vi "datahandle.vi"(8 "error in (no error)":errorcluster caption="错误输入（无错误）", 10 "data":string[][](array[string]), 11 "HJ212 输入":refnum<class "HJ212.lvclass">) -> (0 "error out":errorcluster caption="错误输出", 2 "message":string, 3 "HJ212 输出":refnum<class "HJ212.lvclass">)   [LabVIEW 2016, in "中水三立SQL数据传输.lvlib" / "HJ212.lvclass"]
uses:
  HJ212.lvclass
  data_combination/data_combination.lvclass/data_combination.ctl
  data_combination/data_combination.lvclass
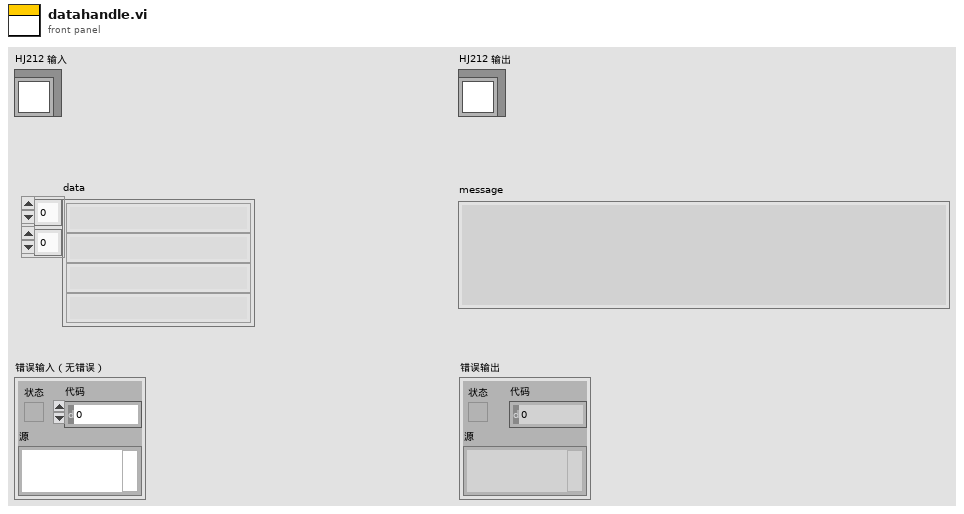
[diagram p1: front panel]
types:
  T1 = cluster{"请求编码QN(20)":string, "系统编码ST(5)":string, "命令编码CN(7)":string, "访问密码PW(9)":string, "设备唯一标识MN(27)":string, "拆分包及应答标志FLAG(8)":string, "总包数PNUM(9)":string, "包号PNO(8)":string, "指令参数CP(0-950)":string}
  T2 = typedef "中水三立SQL数据传输.lvlib/table.ctl" = string
  T3 = typedef "中水三立SQL数据传输.lvlib/Type.ctl" = string
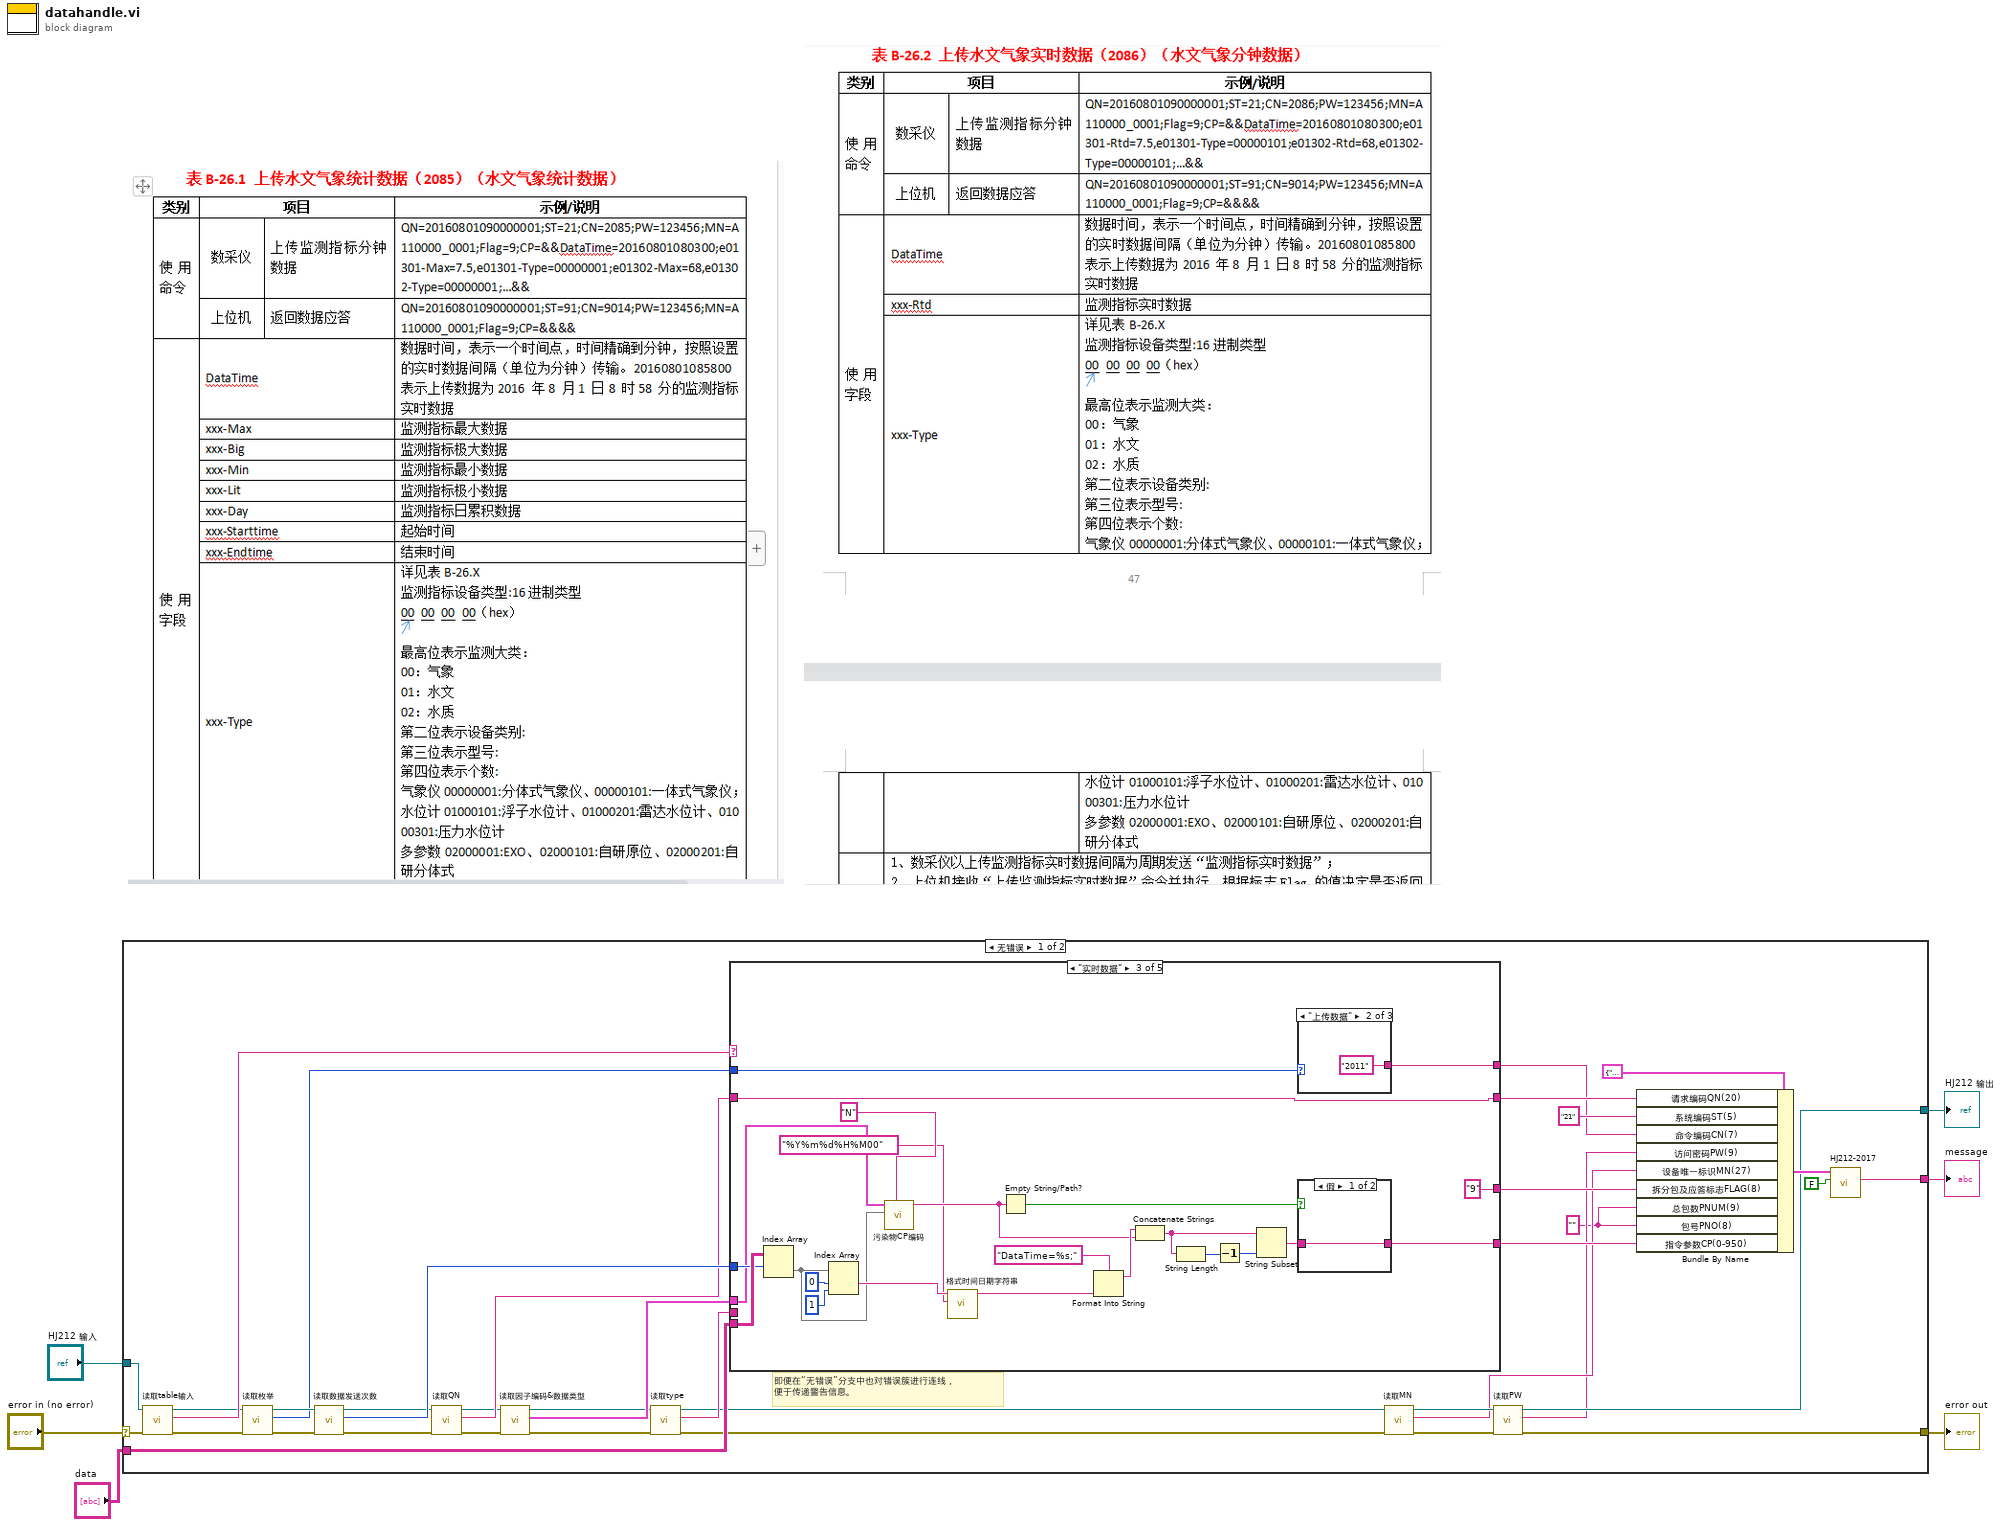
[diagram p0: block diagram]
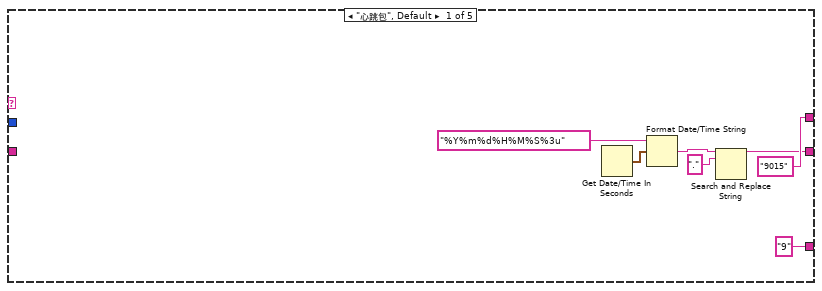
[diagram p2: hidden frame]
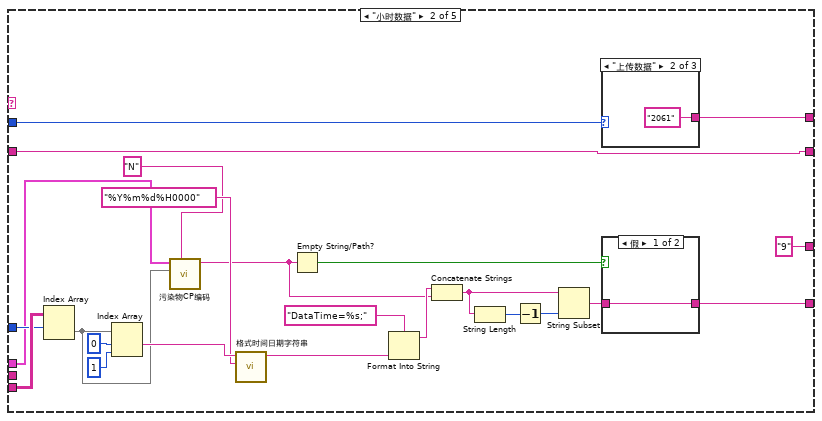
[diagram p3: hidden frame]
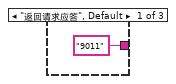
[diagram p4: hidden frame]
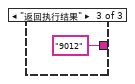
[diagram p5: hidden frame]
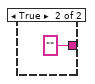
[diagram p6: hidden frame]
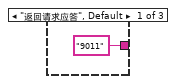
[diagram p7: hidden frame]
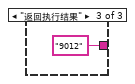
[diagram p8: hidden frame]
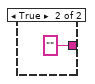
[diagram p9: hidden frame]
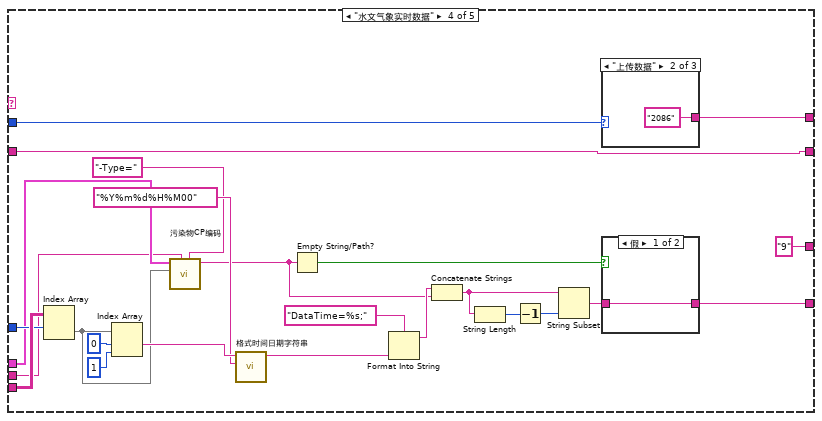
[diagram p10: hidden frame]
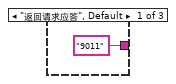
[diagram p11: hidden frame]
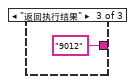
[diagram p12: hidden frame]
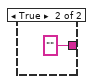
[diagram p13: hidden frame]
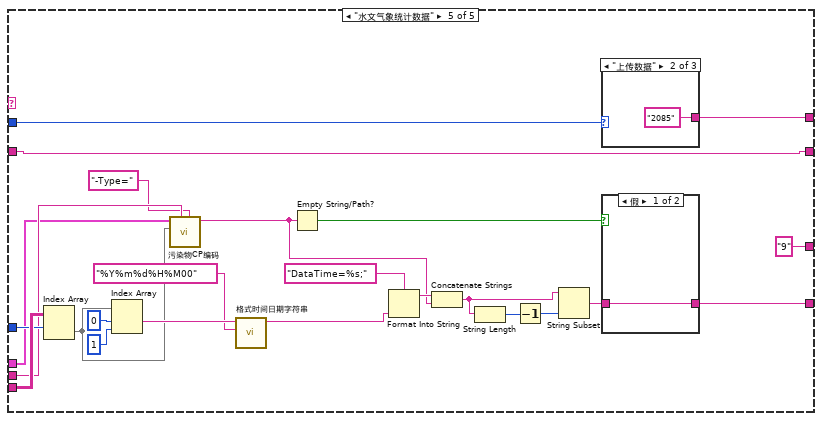
[diagram p14: hidden frame]
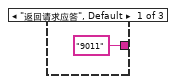
[diagram p15: hidden frame]
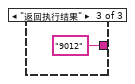
[diagram p16: hidden frame]
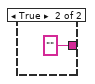
[diagram p17: hidden frame]
diagram:
  n1 = case shown="无错误" "error in (no error)" {
    selector: "error in (no error)" -> [w17 w166]
    tunnel: [w16 w166] -> w5
    tunnel: [w24 w165] -> w3
    tunnel: "HJ212 输入" -> [w26 w165]
    tunnel: [w43 _] -> w2
    tunnel: "data" -> [w36 _]
    frame No Error {
      w15 = "" ("总包数PNUM(9)")
      # "即便在“无错误”分支中也对错误簇进行连线，\n便于传递警告信息。"
      n2 = call "读取table输入.vi"("error in (no error)"=w17, "data_combination输入"=w26) -> ("error out"=w21:errorcluster, "table输入"=w39:T2, "data_combination输出"=w38:refnum<class "HJ212.lvclass">)  [unwired: 7 in]
      n3 = call "读取枚举.vi"("error in (no error)"=w21, "data_combination输入"=w38) -> ("error out"=w20:errorcluster, "枚举"=w28:enum16{"返回请求应答", "上传数据", "返回执行结果"}, "data_combination输出"=w37:refnum<class "HJ212.lvclass">)  [unwired: 7 in]
      n4 = call "读取数据发送次数.vi"("error in (no error)"=w20, "data_combination输入"=w37) -> ("error out"=w19:errorcluster, "数据发送次数"=w35:i32, "data_combination输出"=w31:refnum<class "HJ212.lvclass">)  [unwired: 7 in]
      n5 = call "读取QN.vi"("error in (no error)"=w19, "data_combination输入"=w31) -> ("error out"=w13:errorcluster, "QN"=w30:string, "data_combination输出"=w14:refnum<class "HJ212.lvclass">)  [unwired: 7 in]
      n6 = call "读取因子编码&数据类型.vi"("error in (no error)"=w13, "data_combination输入"=w14) -> ("error out"=w7:errorcluster, "因子编码&数据类型"=w12:cluster{"因子编码":string, "数据类型":string}[], "data_combination输出"=w8:refnum<class "HJ212.lvclass">)  [unwired: 7 in]
      n7 = call "读取type.vi"("error in (no error)"=w7, "data_combination输入"=w8) -> ("error out"=w9:errorcluster, "type"=w11:T3, "data_combination输出"=w10:refnum<class "HJ212.lvclass">)  [unwired: 7 in]
      n8 = case shown="\"实时数据\"" w39 {
        tunnel: w36 -> [_ w72 w100 w129 w143]
        tunnel: w35 -> [_ w71 w99 w128 w140]
        tunnel: [_ w61 w90 w118 w142] -> w34
        tunnel: ["9" ("ST") "9" ("ST") "9" ("ST") "9" ("ST") "9" ("ST")] -> w33
        tunnel: [w46 w59 w88 w116 w144] -> w29
        tunnel: w30 -> [_ w59 w88 w116 w144]
        tunnel: w28 -> [_ w58 w87 w115 w146]
        tunnel: ["9015" ("ST") w57 w86 w114 w145] -> w27
        tunnel: w12 -> [_ w54 w83 w112 w137]
        tunnel: w11 -> [_ _ _ w107 w139]
        frame "心跳包", Default {
          n9 = Get Date/Time In Seconds() -> (seconds since 1Jan1904=w49:timestamp)
          n10 = Format Date/Time String(time format string (%c)="%Y%m%d%H%M%S%3u" ("时间格式字符串(%c)"), seconds (now)=w49) -> (date/time string=w48:string)  [unwired: 1 in]
          n11 = Search and Replace String(input string=w48, search string="." ("搜索字符串")) -> (result string=w46:string)  [unwired: 6 in, 3 out]
        }
        frame "小时数据" {
          n12 = Index Array(array=w72, index (row)=w71) -> (element=w51:string[])  [unwired: 1 in]
          n13 = Index Array(array=w51, index #1=0 ("索引"), index #2=1 ("索引")) -> (element #1=w70:string)  [unwired: 1 out]
          n14 = call "污染物CP编码.vi"("Type/标识"="N" ("字符串"), "污染物浓度"=w51, "因子编码&数据类型"=w54) -> ("编码输出"=w52:string)  [unwired: 8 in]
          n15 = call "格式时间日期字符串.vi"("时间格式字符串(%c)"="%Y%m%d%H0000", "字符串"=w70) -> ("result string"=w67:string)  [unwired: 9 in]
          n16 = Empty String/Path?(string/path=w52) -> (empty?=w53:bool)
          n17 = Format Into String(format string="DataTime=%s;", w67) -> (resulting string=w62:string)  [unwired: 2 in, 1 out]
          n18 = Concatenate Strings(w62, w52) -> (w64:string)
          n19 = String Length(string=w64) -> (length=w66:i32)
          n20 = Decrement(x=w66) -> (x-1=w65:i32)
          n21 = String Subset(string=w64, length (rest)=w65) -> (substring=w63:string)  [unwired: 1 in]
          n22 = case shown="\"上传数据\"" w58 {
            tunnel: ["9011" ("CN") "2061" ("CN") "9012" ("CN")] -> w57
            frame "返回请求应答", Default {
            }
            frame "上传数据" {
            }
            frame "返回执行结果" {
            }
          }
          n23 = case shown="假" w53 {
            tunnel: [w77 ""] -> w61
            tunnel: w63 -> [w77 _]
            frame False {
            }
            frame True {
            }
          }
        }
        frame "实时数据" {
          n24 = Index Array(array=w100, index (row)=w99) -> (element=w80:string[])  [unwired: 1 in]
          n25 = Index Array(array=w80, index #1=0 ("索引"), index #2=1 ("索引")) -> (element #1=w98:string)  [unwired: 1 out]
          n26 = call "污染物CP编码.vi"("Type/标识"="N" ("字符串"), "污染物浓度"=w80, "因子编码&数据类型"=w83) -> ("编码输出"=w81:string)  [unwired: 8 in]
          n27 = call "格式时间日期字符串.vi"("时间格式字符串(%c)"="%Y%m%d%H%M00", "字符串"=w98) -> ("result string"=w96:string)  [unwired: 9 in]
          n28 = Empty String/Path?(string/path=w81) -> (empty?=w82:bool)
          n29 = Format Into String(format string="DataTime=%s;", w96) -> (resulting string=w91:string)  [unwired: 2 in, 1 out]
          n30 = Concatenate Strings(w91, w81) -> (w93:string)
          n31 = String Length(string=w93) -> (length=w95:i32)
          n32 = Decrement(x=w95) -> (x-1=w94:i32)
          n33 = String Subset(string=w93, length (rest)=w94) -> (substring=w92:string)  [unwired: 1 in]
          n34 = case shown="\"上传数据\"" w87 {
            tunnel: ["9011" ("CN") "2011" ("CN") "9012" ("CN")] -> w86
            frame "返回请求应答", Default {
            }
            frame "上传数据" {
            }
            frame "返回执行结果" {
            }
          }
          n35 = case shown="假" w82 {
            tunnel: [w105 ""] -> w90
            tunnel: w92 -> [w105 _]
            frame False {
            }
            frame True {
            }
          }
        }
        frame "水文气象实时数据" {
          n36 = Index Array(array=w129, index (row)=w128) -> (element=w109:string[])  [unwired: 1 in]
          n37 = Index Array(array=w109, index #1=0 ("索引"), index #2=1 ("索引")) -> (element #1=w127:string)  [unwired: 1 out]
          n38 = call "污染物CP编码.vi"("-flag="="-Type=" ("-fag="), "Type/标识"=w107, "污染物浓度"=w109, "因子编码&数据类型"=w112) -> ("编码输出"=w110:string)  [unwired: 7 in]
          n39 = call "格式时间日期字符串.vi"("时间格式字符串(%c)"="%Y%m%d%H%M00", "字符串"=w127) -> ("result string"=w124:string)  [unwired: 9 in]
          n40 = Empty String/Path?(string/path=w110) -> (empty?=w111:bool)
          n41 = Format Into String(format string="DataTime=%s;", w124) -> (resulting string=w119:string)  [unwired: 2 in, 1 out]
          n42 = Concatenate Strings(w119, w110) -> (w121:string)
          n43 = String Length(string=w121) -> (length=w123:i32)
          n44 = Decrement(x=w123) -> (x-1=w122:i32)
          n45 = String Subset(string=w121, length (rest)=w122) -> (substring=w120:string)  [unwired: 1 in]
          n46 = case shown="\"上传数据\"" w115 {
            tunnel: ["9011" ("CN") "2086" ("CN") "9012" ("CN")] -> w114
            frame "返回请求应答", Default {
            }
            frame "上传数据" {
            }
            frame "返回执行结果" {
            }
          }
          n47 = case shown="假" w111 {
            tunnel: [w134 ""] -> w118
            tunnel: w120 -> [w134 _]
            frame False {
            }
            frame True {
            }
          }
        }
        frame "水文气象统计数据" {
          n48 = Index Array(array=w143, index (row)=w140) -> (element=w136:string[])  [unwired: 1 in]
          n49 = Index Array(array=w136, index #1=0 ("索引"), index #2=1 ("索引")) -> (element #1=w158:string)  [unwired: 1 out]
          n50 = call "污染物CP编码.vi"("-flag="="-Type=" ("-fag="), "Type/标识"=w139, "污染物浓度"=w136, "因子编码&数据类型"=w137) -> ("编码输出"=w147:string)  [unwired: 7 in]
          n51 = call "格式时间日期字符串.vi"("时间格式字符串(%c)"="%Y%m%d%H%M00", "字符串"=w158) -> ("result string"=w155:string)  [unwired: 9 in]
          n52 = Empty String/Path?(string/path=w147) -> (empty?=w148:bool)
          n53 = Format Into String(format string="DataTime=%s;", w155) -> (resulting string=w150:string)  [unwired: 2 in, 1 out]
          n54 = Concatenate Strings(w150, w147) -> (w152:string)
          n55 = String Length(string=w152) -> (length=w154:i32)
          n56 = Decrement(x=w154) -> (x-1=w153:i32)
          n57 = String Subset(string=w152, length (rest)=w153) -> (substring=w151:string)  [unwired: 1 in]
          n58 = case shown="\"上传数据\"" w146 {
            tunnel: ["9011" ("CN") "2085" ("CN") "9012" ("CN")] -> w145
            frame "返回请求应答", Default {
            }
            frame "上传数据" {
            }
            frame "返回执行结果" {
            }
          }
          n59 = case shown="假" w148 {
            tunnel: [w163 ""] -> w142
            tunnel: w151 -> [w163 _]
            frame False {
            }
            frame True {
            }
          }
        }
      }
      n60 = call "读取MN.vi"("error in (no error)"=w9, "data_combination输入"=w10) -> ("error out"=w18:errorcluster, "MN"=w23:string, "data_combination输出"=w25:refnum<class "HJ212.lvclass">)  [unwired: 7 in]
      n61 = call "读取PW.vi"("error in (no error)"=w18, "data_combination输入"=w25) -> ("error out"=w16:errorcluster, "PW"=w22:string, "data_combination输出"=w24:refnum<class "HJ212.lvclass">)  [unwired: 7 in]
      n62 = Bundle By Name(cluster=T1 {"请求编码QN(20)"="", "系统编码ST(5)"="", "命令编码CN(7)"="", "访问密码PW(9)"="", "设备唯一标识MN(27)"="", "拆分包及应答标志FLAG(8)"="", "总包数PNUM(9)"="", "包号PNO(8)"="", "指令参数CP(0-950)"=""} ("数据段"), "请求编码QN(20)"=w29, "系统编码ST(5)"="21", "命令编码CN(7)"=w27, "访问密码PW(9)"=w22, "设备唯一标识MN(27)"=w23, "拆分包及应答标志FLAG(8)"=w33, "总包数PNUM(9)"=w15, "包号PNO(8)"=w15, "指令参数CP(0-950)"=w34) -> (w40:T1)
      n63 = call "HJ212-2017.vi"("PWD？"=FALSE, "数据段"=w40) -> ("通讯包字符串"=w43:string)  [unwired: 7 in, 2 out]
    }
    frame Error {
    }
  }
  "error out" <- w5
  "HJ212 输出" <- w3
  "message" <- w2
